vi "LVClass_CameraSet Get Parameter Type.vi"(0 "CameraSet.lvclass":refnum<class "CameraSet.lvclass">, 5 "parameter_name":string, 11 "error in (no error)":errorcluster) -> (4 "CameraSet.lvclass":refnum<class "CameraSet.lvclass">, 6 "Type":T1, 15 "error out":errorcluster)   [LabVIEW 2020, in "CameraSet.lvclass"]
doc: "Camera parameter type getter given its name which should have been read with\nImop_CameraSet_GetParameterName.\n\n<B>camera_setIn</B> : CameraSet object.\n<B>camera_setOut</B> : CameraSet object.\n<B>parameter_name</B> : Parameter name.\n<B>type</B> : Parameter type value, \n See : E_TYPES_T"
uses:
  CameraSet.lvclass
  Controls/CameraParameters_Type.ctl
  CameraSet.lvclass/CameraSet.ctl
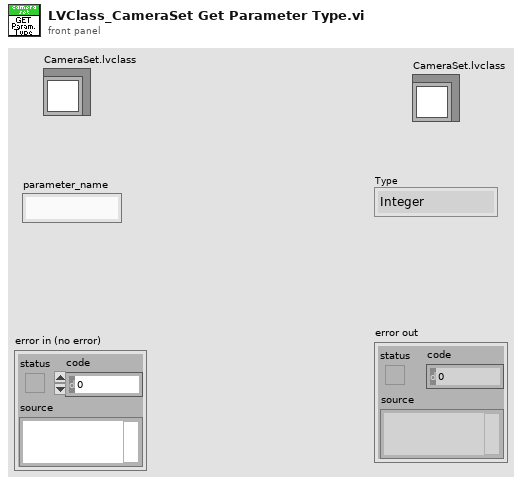
[diagram p1: front panel]
types:
  T1 = typedef "CameraParameters_Type.ctl" = enum16{"Integer", "Real", "String", "Boolean"}
  T2 = typedef "ClassID.ctl" = i64
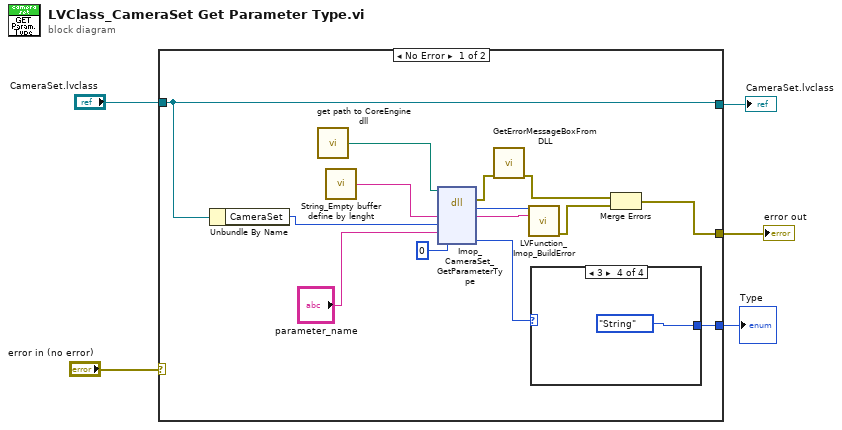
[diagram p0: block diagram]
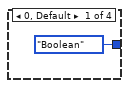
[diagram p2: hidden frame]
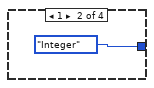
[diagram p3: hidden frame]
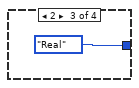
[diagram p4: hidden frame]
diagram:
  n1 = case shown="No Error" "error in (no error)" {
    selector: "error in (no error)" -> [_ w24]
    tunnel: "CameraSet.lvclass" -> [w10 w25]
    tunnel: [w10 w25] -> w3
    tunnel: [w6 w24] -> w2
    tunnel: [w11 _] -> w1
    frame No Error {
      n2 = Unbundle By Name(w10) -> ("CameraSet"=w9:T2)
      n3 = call "get path to CoreEngine dll.vi"() -> ("path to wavekit library"=w14:path)  [unwired: 14 in, 1 out]
      n4 = call "String_Empty buffer define by lenght.vi"() -> ("Empty buffer"=w17:string)  [unwired: 1 in]
      n5 = dll-call lib="D:/2_trunk/temp_core_engine/DLLs/ImopEngine4_vc100.dll" fn="Imop_CameraSet_GetParameterType"(path in=w14, "message"=w17, "objet"=w9, "parameter_name"="parameter_name", "type"=u32 0) -> (error out=w13:errorcluster, "return type"=w19:i32, "message"=w18:string, "type"=w12:i32)  [unwired: 4 in, 1 out]
      n6 = call "GetErrorMessageBoxFromDLL.vi"("error IN"=w13) -> ("error OUT"=w8:errorcluster)  [unwired: 10 in]
      n7 = call "LVFunction_Imop_BuildError.vi"("code"=w19, "String to Prepend to source (\"\")"=w18) -> ("error out"=w7:errorcluster)  [unwired: 13 in]
      n8 = case shown="3" w12 {
        tunnel: [CameraParameters_Type."Boolean" ("Type 2") CameraParameters_Type."Integer" ("Type 2") CameraParameters_Type."Real" ("Type 2") CameraParameters_Type."String" ("Type 2")] -> w11
        frame 0, Default {
        }
        frame 1 {
        }
        frame 2 {
        }
        frame 3 {
        }
      }
      n9 = Merge Errors(w8, w7) -> (w6:errorcluster)
    }
    frame Error {
    }
  }
  "CameraSet.lvclass" <- w3
  "error out" <- w2
  "Type" <- w1
